vi "Turret and Robot Angle Adjust.vi"(6 "Turret field of view":dbl, 8 "Robot start angle reletive to hopper":dbl, 9 "Robot angle":dbl, 10 "Turret start angle reletive to center line or 0":dbl, 11 "Turret angle":dbl) -> (1 "Robot angle to Rotate":dbl, 3 "Turret angle to Rotate":dbl)   [LabVIEW 2016]
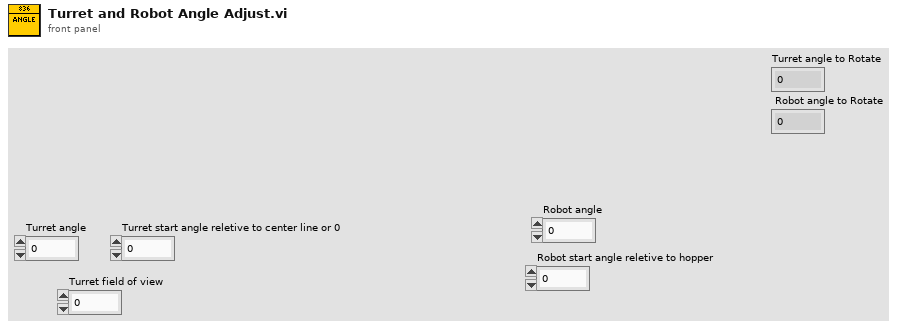
[diagram p1: front panel]
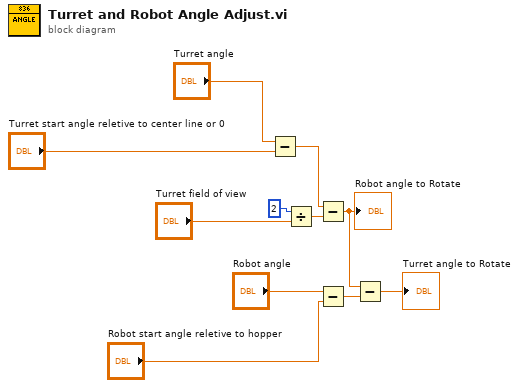
[diagram p0: block diagram]
diagram:
  n1 = Subtract(x="Turret angle", y="Turret start angle reletive to center line or 0") -> (x-y=w11:dbl)
  n2 = Divide(x=2, y="Turret field of view") -> (x/y=w9:dbl)
  n3 = Subtract(x=w11, y=w9) -> (x-y=w6:dbl)
  "Robot angle to Rotate" <- w6
  n4 = Subtract(x="Robot angle", y="Robot start angle reletive to hopper") -> (x-y=w8:dbl)
  n5 = Subtract(x=w6, y=w8) -> (x-y=→"Turret angle to Rotate":dbl)
